vi "Usrednianie wektora.vi"(7 "length (10)":i32=10, 11 "Array in":dbl[](array[numeric])) -> (3 "Array out":dbl[](array[numeric]))   [LabVIEW 2014]
doc: "Uśrednia wartości wejściowe obliczając średnią biegnącą\nz pamięcią length (10) ostatnich próbek poprzedniego wektora"
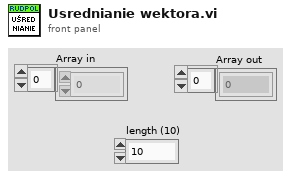
[diagram p1: front panel]
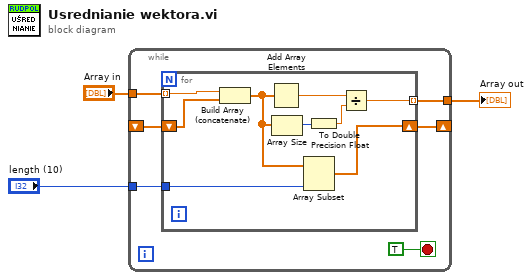
[diagram p0: block diagram]
diagram:
  n1 = while {
    tunnel: "length (10)" -> [w8]
    shift-right: [w5] -> _
    shift-left: _ -> [w4]
    tunnel: "Array in" -> [w9]
    tunnel: [w7] -> w3
    stop <- TRUE stop-if-true
    n2 = for {
      tunnel: w9 -> [w18] mode=indexing
      tunnel: w8 -> [w13]
      shift-right: [w10] -> w5
      shift-left: w4 -> [w12]
      tunnel: [w11] -> w7 mode=indexing
      n3 = Build Array (concatenate)(w18, w12) -> (w14:dbl[])
      n4 = Add Array Elements(numeric array=w14) -> (sum=w17:dbl)
      n5 = Array Size(array=w14) -> (size(s)=w16:i32)
      n6 = Array Subset(array=w14, length=w13) -> (w10:dbl[])  [unwired: 1 in]
      n7 = To Double Precision Float(number=w16) -> (double precision float=w15:dbl)
      n8 = Divide(x=w17, y=w15) -> (x/y=w11:dbl)
    }
  }
  "Array out" <- w3
